vi "Launcher.vi"(8 "error in (no error)":errorcluster, 10 "TopLevel":refnum<class "TopLevel.lvclass">, 11 "DLP2 in":refnum<class "DLP2.lvclass">) -> (0 "error out":errorcluster, 3 "DLP2 out":refnum<class "DLP2.lvclass">)   [LabVIEW 2022 SP3, in "DLP2.lvclass"]
uses:
  DLP2.lvclass
  TopLevel/TopLevel.lvclass
  Process.vi
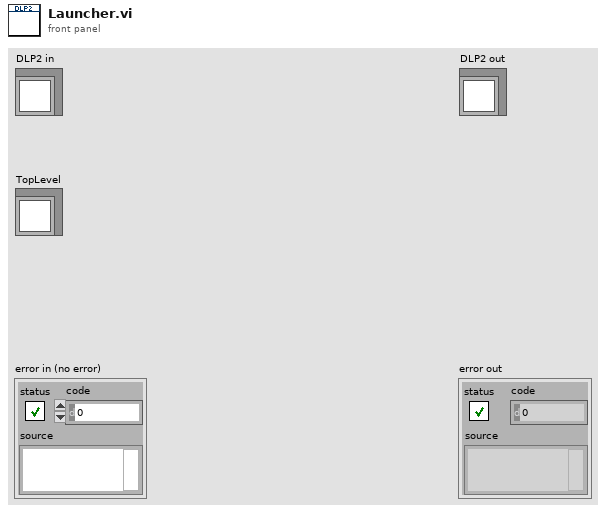
[diagram p1: front panel]
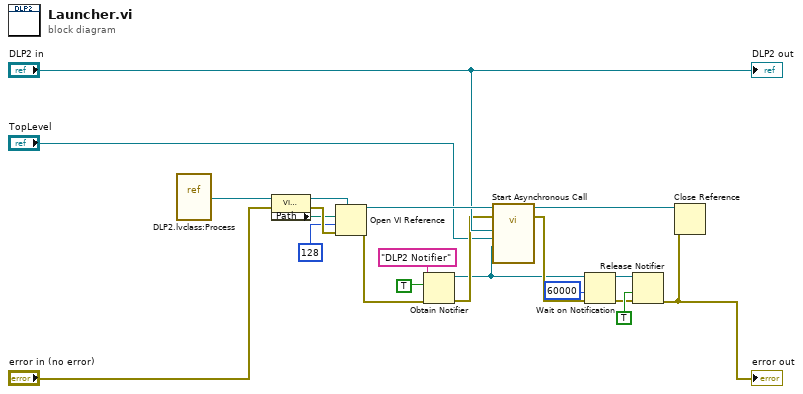
[diagram p0: block diagram]
diagram:
  n1 = vi-ref "DLP2.lvclass:Process.vi"() -> (w7:refnum<vi>)
  n2 = property class="VI (strict)"(reference=w7, error in="error in (no error)") -> (reference out=w9:refnum<vi>, error out=w15:errorcluster, "Path"=w8:path)
  n3 = Open VI Reference(type specifier VI Refnum (for type only)=w9, vi path=w8, options=128, error in (no error)=w15) -> (vi reference=w11:refnum<vi>, error out=w14:errorcluster)  [unwired: 2 in]
  n4 = Obtain Notifier(name (unnamed)="DLP2 Notifier", notification data type=TRUE, error in (no error)=w14) -> (notifier out=w1:refnum<notifier>, error out=w3:errorcluster)  [unwired: 1 in, 1 out]
  n5 = call-by-ref "Start Asynchronous Call"(reference=w11, error in=w3, "process sync"=w1, "TopLevel"="TopLevel", "DLP2 in"="DLP2 in") -> (reference out=w19:refnum<vi>, error out=w13:errorcluster)  [unwired: 9 in]
  n6 = Wait on Notification(notifier=w1, timeout in ms (-1)=60000, error in (no error)=w13) -> (notifier out=w18:refnum<notifier>, error out=w17:errorcluster)  [unwired: 1 in, 2 out]
  n7 = Release Notifier(notifier=w18, force destroy? (F)=TRUE, error in (no error)=w17) -> (error out=w5:errorcluster)  [unwired: 2 out]
  "error out" <- w5
  n8 = Close Reference(reference=w19, error in (no error)=w5) -> ()  [unwired: 1 out]
  "DLP2 out" <- "DLP2 in"
